vi "Add_Color.vi"(9 "Color":T1 items=["Automatic"=2147483647, "Black"=0, "White"=16777215, "Red"=16711680, "Green"=2263842, "Blue"=255, "Cyan"=65535, "Magenta"=16711935, "Yellow"=16776960], 10 "Key":string, 11 "Keyword Array":T2[](array[typedef])) -> (3 "Keyword Array Out":T2[](array[typedef]))   [LabVIEW 2013, in "Advanced Plotting Toolkit.lvlib"]
uses:
  Advanced Plotting Toolkit.lvlib
  KeyValue.ctl
  typedefs/PlotColor.ctl
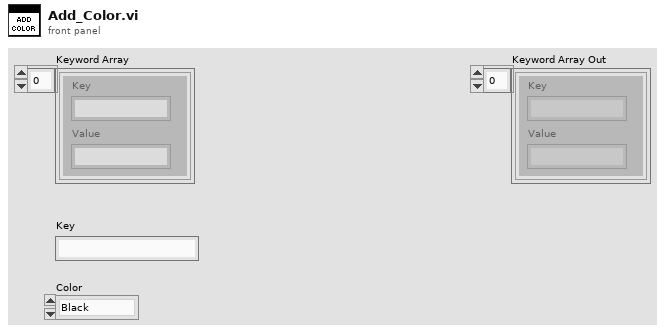
[diagram p1: front panel]
types:
  T1 = typedef "Advanced Plotting Toolkit.lvlib/PlotColor.ctl" = u32
  T2 = typedef "Advanced Plotting Toolkit.lvlib/KeyValue.ctl" = cluster{"Key":string, "Value":string}
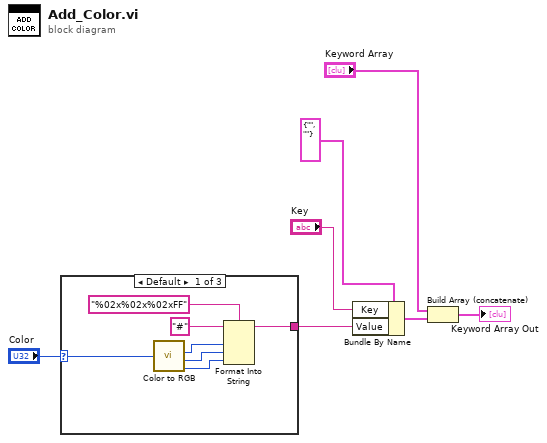
[diagram p0: block diagram]
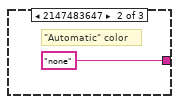
[diagram p2: hidden frame]
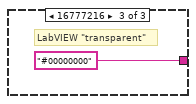
[diagram p3: hidden frame]
diagram:
  n1 = case shown="Default" "Color" {
    selector: "Color" -> [w14 _ _]
    tunnel: [w9 "none" ("f") "#00000000"] -> w1
    frame Default {
      n2 = call <vilib>:"Color to RGB.vi"("Color"=w14) -> ("R"=w8:u8, "G"=w11:u8, "B"=w10:u8)  [unwired: 1 out]
      n3 = Format Into String(format string="%02x%02x%02xFF", initial string="#", w8, w11, w10) -> (resulting string=w9:string)  [unwired: 1 in, 1 out]
    }
    frame 2147483647 {
      # "\"Automatic\" color"
    }
    frame 16777216 {
      # "LabVIEW \"transparent\""
    }
  }
  n4 = Bundle By Name(cluster=T2 {"Key"="", "Value"=""} ("KeyValue"), "Key"="Key", "Value"=w1) -> (w5:T2)
  n5 = Build Array (concatenate)("Keyword Array", w5) -> (→"Keyword Array Out":T2[])
